vi "gjson_Create.vi"(8 "error in":errorcluster, 11 "JSON Object in":variant) -> (0 "error out":errorcluster, 3 "JSON String Out":string)   [LabVIEW 2015, in "Json2Labv.lvlib"]
uses:
  Json2Labv.lvlib
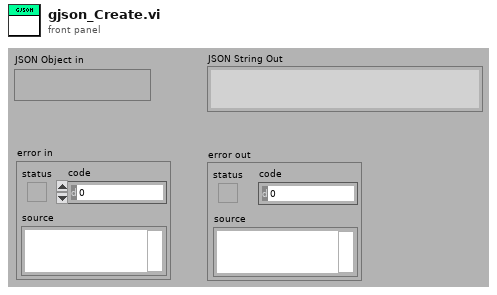
[diagram p1: front panel]
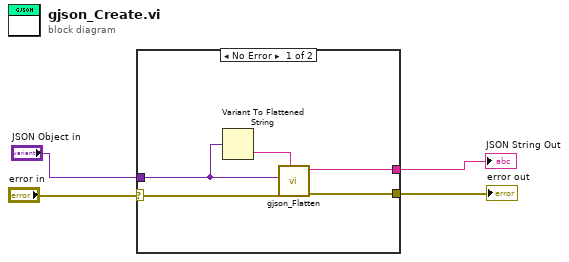
[diagram p0: block diagram]
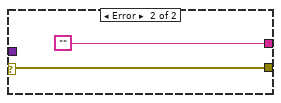
[diagram p2: hidden frame]
diagram:
  n1 = case shown="No Error" "error in" {
    selector: "error in" -> [w9 w10]
    tunnel: "JSON Object in" -> [w7 _]
    tunnel: [w6 w10] -> w1
    tunnel: [w5 ""] -> w2
    frame No Error {
      n2 = Variant To Flattened String(Variant=w7) -> (data string=w8:string)  [unwired: 1 out]
      n3 = call "gjson_Flatten.vi"("FlattenedData"=w8, "error in"=w9, "Variant"=w7) -> ("error out"=w6:errorcluster, "JSON String Out"=w5:string)  [unwired: 6 in, 1 out]
    }
    frame Error {
    }
  }
  "JSON String Out" <- w2
  "error out" <- w1
